vi "Reset.vi"(8 "error in (no error)":errorcluster, 11 "VISA resource name":refnum<visa-resource-name>) -> (0 "error out":errorcluster, 3 "VISA resource name out":refnum<visa-resource-name>)   [LabVIEW 2019, in "Andeen-Hagerling 2700(400 firmware).lvlib"]
doc: "Puts all measurement circuitry and all higher control sections of the bridge except for the bus control circuitry into the same state as at power-on then sends a set of default setup commands to the instrument."
uses:
  Andeen-Hagerling 2700(400 firmware).lvlib
  <vilib>/Instr/_visa.llb/VISA Flush IO Buffer Mask.ctl
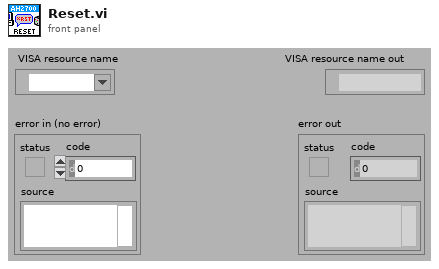
[diagram p1: front panel]
types:
  T1 = typedef "VISA Flush IO Buffer Mask.ctl" = u16
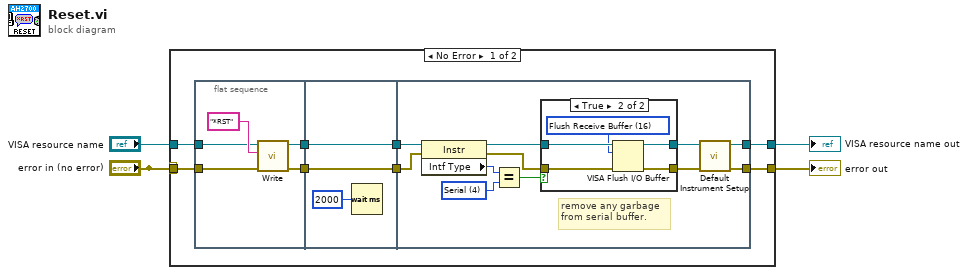
[diagram p0: block diagram]
diagram:
  n1 = case shown="No Error" "error in (no error)" {
    selector: "error in (no error)" -> [w7 w40]
    tunnel: "error in (no error)" -> [_ _]
    tunnel: "VISA resource name" -> [w8 w39]
    tunnel: [w6 w39] -> w3
    tunnel: [w5 w40] -> w2
    frame No Error {
      n2 = flat-sequence {
        tunnel: w8 -> [w16]
        tunnel: w7 -> [w15]
        tunnel: [w14] -> w12
        tunnel: [w13] -> w11
        tunnel: w12 -> [w18]
        tunnel: w11 -> [w19]
        tunnel: [w19] -> w10
        tunnel: [w18] -> w9
        tunnel: w10 -> [w23]
        tunnel: w9 -> [w24]
        tunnel: [w22] -> w6
        tunnel: [w21] -> w5
        frame #0 {
          n3 = call "Write.vi"("error in"=w15, "command"="*RST" ("Reset Command"), "VISA resource name"=w16) -> ("error out"=w13:errorcluster, "VISA resource name out"=w14:refnum<visa-resource-name>)  [unwired: 7 in]
        }
        frame #1 {
          n4 = Wait (ms)(milliseconds to wait=u32 2000) -> ()  [unwired: 1 out]
        }
        frame #2 {
          w25 = u16 4 items=["GPIB"=1, "VXI"=2, "GPIB-VXI"=3, "Serial"=4, "PXI"=5, "TCPIP"=6, "USB"=7, "FireWire"=9] ("Interface Information:Interface Type")
          # "remove any garbage\nfrom serial buffer."
          n5 = property class="Instr"(reference=w24, error in=w23) -> (reference out=w28:refnum<visa-resource-name>, error out=w29:errorcluster, "Intf Type"=w26:u16)
          n6 = Equal?(x=w26, y=w25) -> (x = y?=w31:bool)
          n7 = case shown="True" w31 {
            tunnel: [w33 w38] -> w27
            tunnel: w28 -> [w33 w37]
            tunnel: w29 -> [w32 w36]
            tunnel: [w32 w35] -> w30
            frame False {
            }
            frame True {
              w34 = T1 16 items=["Flush Receive Buffer"=16, "Write Transmit Buffer to Device"=32, "Flush Receive Buffer (No I/O)"=64, "Flush Transmit Buffer"=128] ("Mask")
              n8 = VISA Flush I/O Buffer(VISA resource name=w37, mask (16)=w34, error in (no error)=w36) -> (VISA resource name out=w38:refnum<visa-resource-name>, error out=w35:errorcluster)
            }
          }
          n9 = call "Default Instrument Setup.vi"("error in (no error)"=w30, "VISA resource name"=w27) -> ("error out"=w21:errorcluster, "VISA resource name out"=w22:refnum<visa-resource-name>)  [unwired: 8 in]
        }
      }
    }
    frame Error {
    }
  }
  "error out" <- w2
  "VISA resource name out" <- w3
